vi "RotateAround2.vi"(6 "Centre":dbl[](array[numeric])=[-2480.0576171875, -1961.996337890625], 8 "Target":dbl[](array[numeric])=[-2336.5934560704363, -2101.3449456159165], 11 "Position":dbl[](array[numeric])=[-2372.455078125, -2038.0294189453125, 2.456908941268921]) -> (3 "Output\nVelocity":dbl[](array[numeric])=[-0.06847630442095567, 0.015600616492653974, 0.6953495299566059] format="%.2f")   [LabVIEW 2016]
uses:
  <vilib>/Analysis/coordinate.llb/Wrap Angle (scalar).vi
  <vilib>/Analysis/coordinate.llb/2D Cartesian Coordinate Rotation (Scalar).vi
  <vilib>/addons/control/pid/pid.llb/PID (DBL Array).vi
  <vilib>/addons/control/pid/NI_PID_pid.lvlib
  <vilib>/Analysis/NI_AALPro.lvlib
  <vilib>/Analysis/NI_AAL_Angle.lvlib
panel:
  in  "reinitialize? (F)":bool
  in  "output range":cluster{"output high":dbl, "output low":dbl}[](array[cluster])=[{"output high"=3.0, "output low"=-3.0}, {"output high"=3.0, "output low"=-3.0}, {"output high"=6.0, "output low"=-6.0}] {"output low" format="%.2f"; "output high" format="%.2f"}
  in  "PID gains":T1(array[cluster])=[{"proportional gain (Kc)"=0.001, "integral time (Ti, min)"=0.0, "derivative time (Td, min)"=0.0002}, {"proportional gain (Kc)"=0.001, "integral time (Ti, min)"=0.0, "derivative time (Td, min)"=0.0002}, {"proportional gain (Kc)"=10.0, "integral time (Ti, min)"=0.0, "derivative time (Td, min)"=0.0}]
  # "x centre"
  # "y centre"
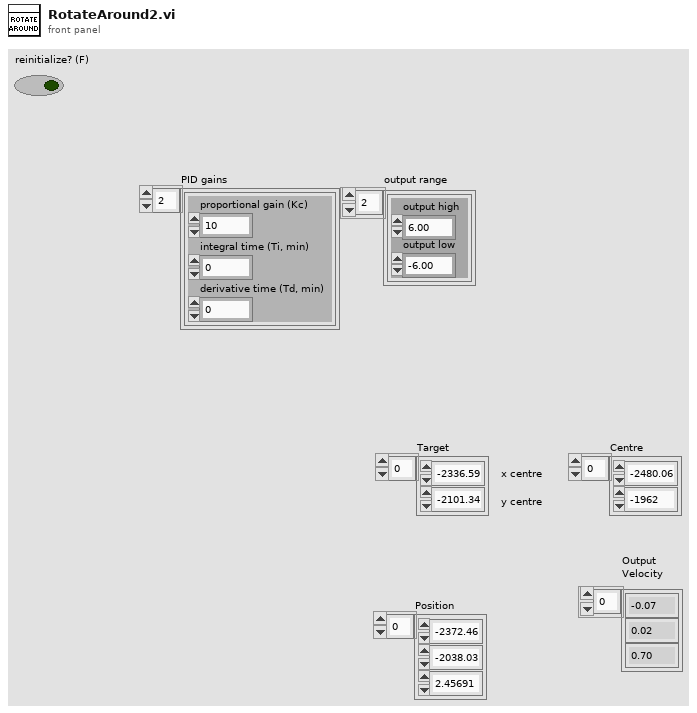
[diagram p1: front panel]
types:
  T1 = cluster{"proportional gain (Kc)":dbl, "integral time (Ti, min)":dbl, "derivative time (Td, min)":dbl}[]
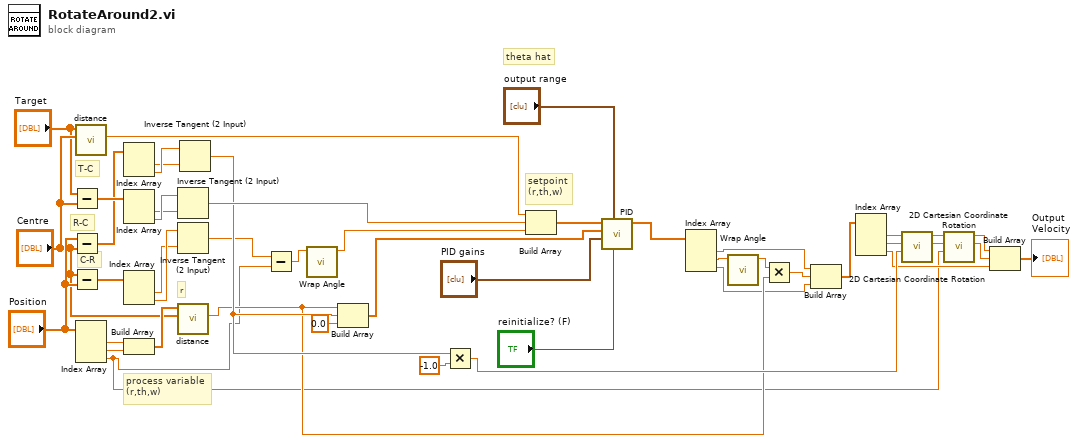
[diagram p0: block diagram]
diagram:
  # "process variable\n(r,th,w)"
  # "setpoint\n(r,th,w)"
  # "r"
  # "C-R"
  # "theta hat"
  # "R-C"
  # "T-C"
  n1 = Subtract(x="Target", y="Centre") -> (x-y=w46:dbl[])
  n2 = Subtract(x="Position", y="Centre") -> (x-y=w41:dbl[])
  n3 = Subtract(x="Centre", y="Position") -> (x-y=w38:dbl[])
  n4 = call "distance.vi"("target pos"="Centre", "obj pos"="Target") -> ("sqrt(x)"=w18:dbl)  [unwired: 9 in]
  n5 = Index Array(array="Position") -> (element #1=w6:dbl, element #2=w40:dbl, element #3=w4:dbl)  [unwired: 3 in]
  n6 = Index Array(array=w41) -> (element #1=w42:dbl, element #2=w43:dbl)  [unwired: 2 in]
  n7 = Index Array(array=w46) -> (element #1=w44:dbl, element #2=w45:dbl)  [unwired: 2 in]
  n8 = Index Array(array=w38) -> (element #1=w36:dbl, element #2=w37:dbl)  [unwired: 2 in]
  n9 = Build Array(w6, w40) -> (w39:dbl[])
  n10 = Inverse Tangent (2 Input)(1:w44, 2:w45) -> (0:w17:dbl)
  n11 = Inverse Tangent (2 Input)(1:w36, 2:w37) -> (0:w5:dbl)
  n12 = call "distance.vi"("target pos"="Centre", "obj pos"=w39) -> ("sqrt(x)"=w12:dbl)  [unwired: 9 in]
  n13 = Inverse Tangent (2 Input)(1:w42, 2:w43) -> (0:w16:dbl)
  n14 = Subtract(x=w5, y=w4) -> (x-y=w2:dbl)
  n15 = call-poly <vilib>:"Wrap Angle.vi"("angle in"=w2) -> ("angle out"=w1:dbl)  [unwired: 9 in, 1 out]
  n16 = Build Array(w12, w16, 0.0 ("element")) -> (w34:dbl[])
  n17 = Multiply(x=w16, y=-1.0) -> (x*y=w30:dbl)
  n18 = Build Array(w18, w17, w1) -> (w35:dbl[])
  n19 = call-poly <vilib>:"PID.vi"("reinitialize? (F)"="reinitialize? (F)", "output range"="output range", "PID gains"="PID gains", "process variable"=w34, "setpoint"=w35) -> ("output"=w15:dbl[])  [unwired: 5 in, 1 out]
  n20 = Index Array(array=w15) -> (element #1=w10:dbl, element #2=w14:dbl, element #3=w9:dbl)  [unwired: 3 in]
  n21 = call-poly <vilib>:"Wrap Angle.vi"("angle in"=w14) -> ("angle out"=w13:dbl)  [unwired: 9 in, 1 out]
  n22 = Multiply(x=w13, y=w12) -> (x*y=w11:dbl)
  n23 = Build Array(w10, w11, w9) -> (w8:dbl[])
  n24 = Index Array(array=w8) -> (element #1=w29:dbl, element #2=w28:dbl, element #3=w22:dbl)  [unwired: 3 in]
  n25 = call-poly <vilib>:"2D Cartesian Coordinate Rotation.vi"("theta"=w30, "y"=w28, "x"=w29) -> ("y out"=w25:dbl, "x out"=w26:dbl)  [unwired: 6 in, 1 out]
  n26 = call-poly <vilib>:"2D Cartesian Coordinate Rotation.vi"("theta"=w4, "y"=w25, "x"=w26) -> ("y out"=w23:dbl, "x out"=w24:dbl)  [unwired: 6 in, 1 out]
  n27 = Build Array(w24, w23, w22) -> (→"Output\nVelocity":dbl[])
